vi "Dictionary Update__ogtk.vi"   [LabVIEW 2012]
doc: "Updates a key-value pair within the dictionary. If the key does not exist, then it will be added to the dictionary, and the created new? output will be TRUE\n\n<B>unlock dictionary</B> (if available on the polymorphic member) will unlock a previously locked dictionary. Locking a dictionary is useful when the values of keys store compound data, which might be modified in multiple locations.\n\nThis polymorphic VI can write a single element or an entire dictionary by value or by reference."
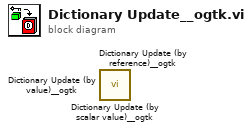
[diagram p0: block diagram]
diagram:
  n1 = call <userlib>:"Dictionary Update (by scalar value)__ogtk.vi"() -> ()  [unwired: 9 in, 3 out]
  n2 = call <userlib>:"Dictionary Update (by reference)__ogtk.vi"() -> ()  [unwired: 9 in, 3 out]
  n3 = call <userlib>:"Dictionary Update (by value)__ogtk.vi"() -> ()  [unwired: 9 in, 3 out]
